vi "waypoint_sensor.vi"(4 "error in":errorcluster, 7 "Waypoint sensor configuration":string="{\n    \"type\": \"Waypoint\",\n    \"listen_port\": 8556,\n    \"debug_tags\": [\"ego\"],\n    \"distance\": 1000.0,\n    \"frequency\": 100.0,\n    \"draw_debug\": false\n}") -> (0 "error out":errorcluster, 1 "Waypoint sensor configuration":string, 3 "Waypoint sensor sample":string)   [LabVIEW 2019, in "Lib_Simx.lvlib"]
doc: "Configure and read the Waypoint sensor information. The waypoint sensor returns a JSON string with information on the waypoints behind and in front of all the actors in the scenario, given the specified distance and frequency. Information about the left and right lanes is also included."
uses:
  Lib_Simx.lvlib
  tools/simx_common.vi
  controls/Header.ctl
panel:
  out "Header":T1 {"game_time" format="%#_9g"}
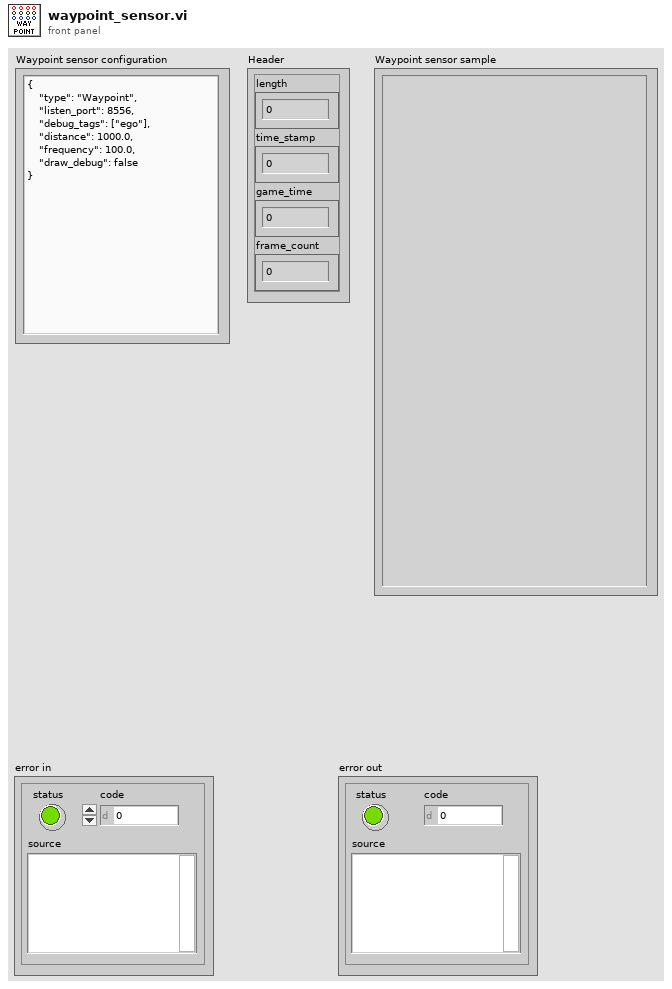
[diagram p1: front panel]
types:
  T1 = typedef "Lib_Simx.lvlib/Header.ctl" = cluster{"length":u32, "time_stamp":u32, "game_time":sgl, "frame_count":u32}
  T2 = typedef "Lib_Simx.lvlib/simx_connection.ctl" = cluster{"Config":T3, "Connections":T6, "Map":cluster{"lanes":cluster{"x":dbl[], "y":dbl[], "z":dbl[]}, "StartPosition":cluster{"start_points":T7, "StartRotation":dbl[], "StartLocation":dbl[]}, "Draw Map Size":T8, "DrawArea":cluster{"min_Y":dbl, "min_X":dbl, "Scale X":dbl, "Scale Y":dbl}, "Map":picture, "Map Geojson":string}}
  T3 = typedef "Lib_Simx.lvlib/config.ctl" = cluster{"Trajectory":T4, "Weather":T5}
  T4 = typedef "Lib_Simx.lvlib/trajectory.ctl" = cluster{"Number of frames":i32, "Frame number":i32, "Trajectory":string}
  T5 = typedef "Lib_Simx.lvlib/weather.ctl" = cluster{"id":string}
  T6 = typedef "Lib_Simx.lvlib/connections.ctl" = cluster{"Simulator Connection":refnum<k5>, "server_ip":string, "Port":i32, "Sensor connections":refnum<k5>[]}
  T7 = typedef "Lib_Simx.lvlib/start_points.ctl" = cluster{"locations":dbl[][], "rotations":dbl[][], "type":string[]}
  T8 = typedef "LVBoundsTypeDef.ctl" = cluster{"Width":u32, "Height":u32}
  T9 = typedef "Lib_Simx.lvlib/sensor_sample.ctl" = cluster{"Header":T1, "data out":string}
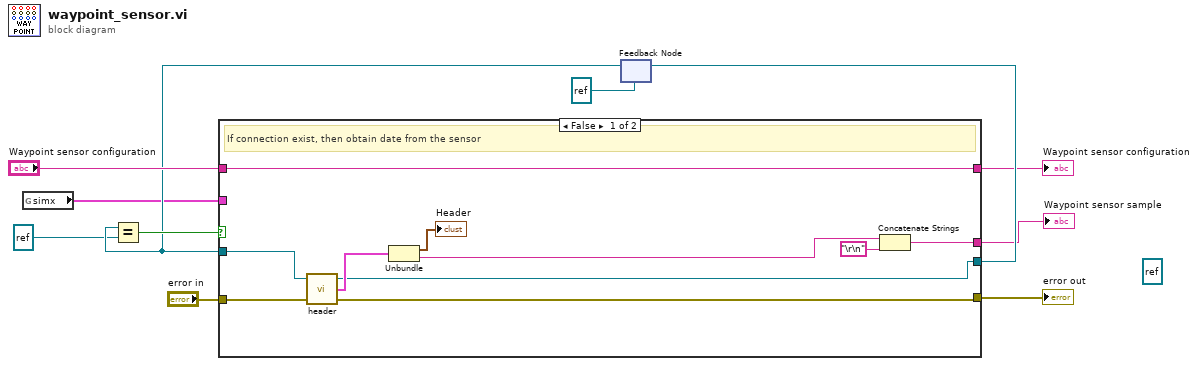
[diagram p0: block diagram]
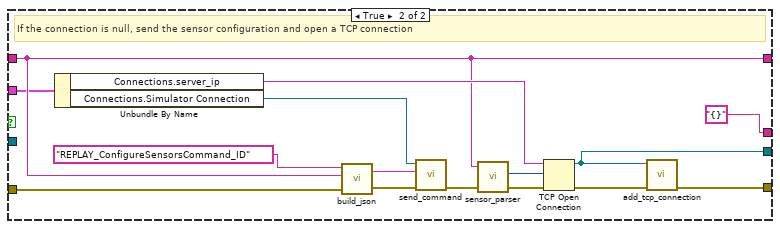
[diagram p2: hidden frame]
diagram:
  (unwired) refnum<k5> refnum ("state_connection")
  n1 = global read "simx_common.vi" "simx"() -> (w3:T2)
  n2 = feedback #1(refnum<k5> refnum ("state_connection")) -> (w7:refnum<k5>)
  n3 = Equal?(x=w7, y=refnum<k5> refnum ("null connection")) -> (x = y?=w8:bool)
  n4 = case shown="False" w8 {
    tunnel: [w17 w25] -> w11
    tunnel: "Waypoint sensor configuration" -> [w16 w27]
    tunnel: [w18 w24] -> w9
    tunnel: w7 -> [w21 _]
    tunnel: "error in" -> [w20 w31]
    tunnel: [w16 w27] -> w5
    tunnel: [w12 "{}" ("data out")] -> w4
    tunnel: w3 -> [_ w23]
    frame False {
      # "If connection exist, then obtain date from the sensor"
      n5 = call "header.vi"("error in"=w20, "TCP Network Connection in"=w21) -> ("error out"=w17:errorcluster, "Sensor sample"=w19:T9, "TCP Network Connection out"=w18:refnum<k5>)  [unwired: 1 in]
      n6 = Unbundle(w19) -> ("Header"=→"Header":T1, "data out"=w13:string)
      n7 = Concatenate Strings(w13, "\r\n") -> (w12:string)
    }
    frame True {
      # "If the connection is null, send the sensor configuration and open a TCP connection"
      n8 = Unbundle By Name(w23) -> ("Connections.server_ip"=w29:string, "Connections.Simulator Connection"=w30:refnum<k5>)
      n9 = call "build_json.vi"("error in"=w31, "Message"=w27, "Command_ID"="REPLAY_ConfigureSensorsCommand_ID") -> ("error out"=w34:errorcluster, "JSON Out"=w35:string)  [unwired: 1 in]
      n10 = call "send_command.vi"("error in"=w34, "JSON Command"=w35, "TCP Network Connection in"=w30) -> ("error out"=w33:errorcluster)  [unwired: 1 in, 3 out]
      n11 = call "sensor_parser.vi"("Sensor configuration"=w27, "error in"=w33) -> ("Port out"=w26:u16, "error out"=w28:errorcluster)  [unwired: 1 in, 2 out]
      n12 = TCP Open Connection(address=w29, remote port or service name=w26, error in (no error)=w28) -> (connection ID=w24:refnum<k5>, error out=w32:errorcluster)  [unwired: 2 in]
      n13 = call "add_tcp_connection.vi"("error in"=w32, "Sensor connection"=w24) -> ("error out"=w25:errorcluster)  [unwired: 5 in]
    }
  }
  "error out" <- w11
  "Waypoint sensor sample" <- w4
  "Waypoint sensor configuration" <- w5
  n14 = feedback-in #1(w9) -> ()
